vi "Increment Time (seconds).vi"(8 "error in (no error)":errorcluster, 10 "nanos offset":i64, 11 "seconds in":dbl) -> (0 "error out":errorcluster, 3 "seconds out":dbl)   [LabVIEW 2013, in "Linux RT Utilities.lvlib"]
doc: "This VI increments the provided timespec by a number of nanoseconds."
uses:
  Linux RT Utilities.lvlib
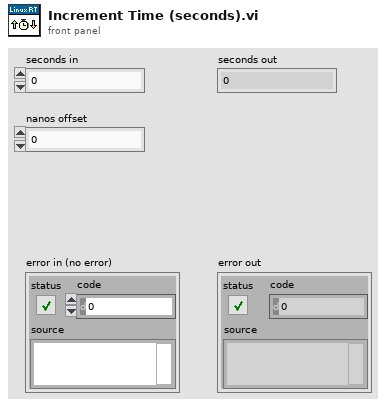
[diagram p1: front panel]
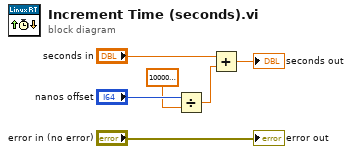
[diagram p0: block diagram]
diagram:
  n1 = Divide(x="nanos offset", y=1000000000.0) -> (x/y=w3:dbl)
  n2 = Add(x="seconds in", y=w3) -> (x+y=→"seconds out":dbl)
  "error out" <- "error in (no error)"
